vi "Dummy Actor Method.vi"(8 "error in (no error)":errorcluster, 11 "Actor in":refnum<class "Actor.lvclass">) -> (0 "error out":errorcluster, 3 "Actor out":refnum<class "Actor.lvclass">)   [LabVIEW 2014, in "original Template.lvlib"]
uses:
  <vilib>/ActorFramework/Actor/Actor.lvclass
  original Template.lvlib
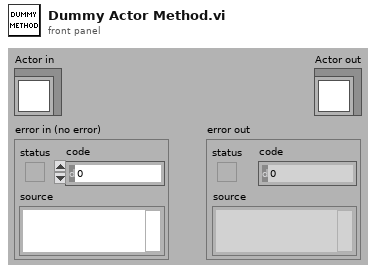
[diagram p1: front panel]
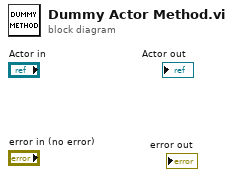
[diagram p0: block diagram]
diagram:
